vi "Sine Waves.vi"() -> ()   [LabVIEW 2010]
uses:
  <vilib>/measure/NI_MABase.lvlib
panel:
  out "System Waveform Graph":waveform(dbl)[](graph)=[{"t0"=timestamp(0 s since 1904-01-01), "dt"=0.001, "Y"=array[250 elements]}, {"t0"=timestamp(0.25 s since 1904-01-01), "dt"=0.001, "Y"=array[250 elements]}, {"t0"=timestamp(0.5 s since 1904-01-01), "dt"=0.001, "Y"=array[250 elements]}, {"t0"=timestamp(0.75 s since 1904-01-01), "dt"=0.001, "Y"=array[250 elements]}]
  # "Sine Waves!"
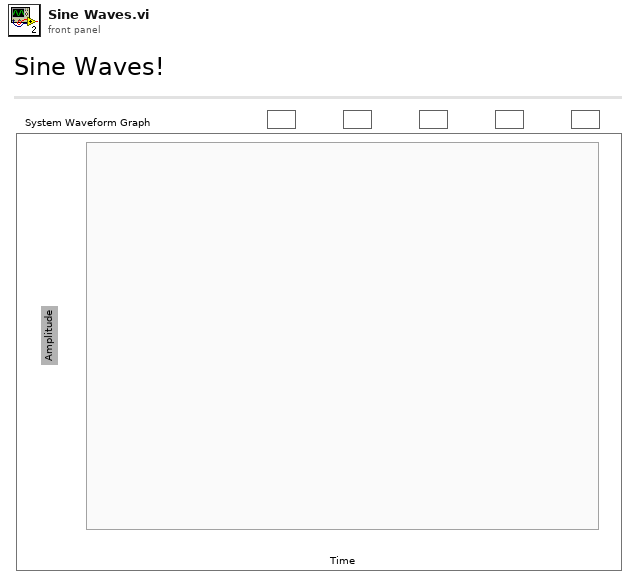
[diagram p1: front panel]
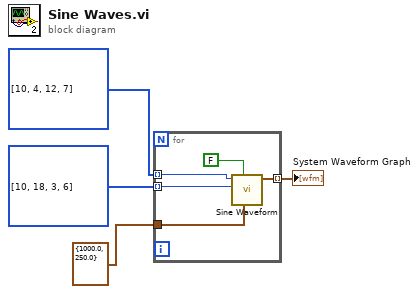
[diagram p0: block diagram]
diagram:
  n1 = for {
    tunnel: i32[] [10, 4, 12, 7] -> [w9] mode=indexing
    tunnel: i32[] [10, 18, 3, 6] -> [w8] mode=indexing
    tunnel: [w7] -> w1 mode=indexing
    tunnel: cluster{"Fs":dbl, "#s":dbl} {"Fs"=1000.0, "#s"=250.0} ("sampling info") -> [w6]
    n2 = call <vilib>:"Sine Waveform.vi"("sampling info"=w6, "reset signal"=FALSE, "amplitude"=w8, "frequency"=w9) -> ("signal out"=w7:waveform(dbl))  [unwired: 6 in, 1 out]
  }
  "System Waveform Graph" <- w1
